vi "Test_PromoteElementAtTop_NoChange.vi"(8 "error in (no error)":errorcluster, 11 "TestCase in":refnum<class "TestArrayExtensions.lvclass">) -> (0 "error out":errorcluster, 3 "TestCase out":refnum<class "TestArrayExtensions.lvclass">)   [LabVIEW 2015, in "TestArrayExtensions.lvclass"]
uses:
  TestArrayExtensions.lvclass
  Promote Element (I32).vi
  <vilib>/addons/_JKI Toolkits/VI Tester/TestCase.llb/TestCase.lvclass
  ArrayExtensions.lvlib
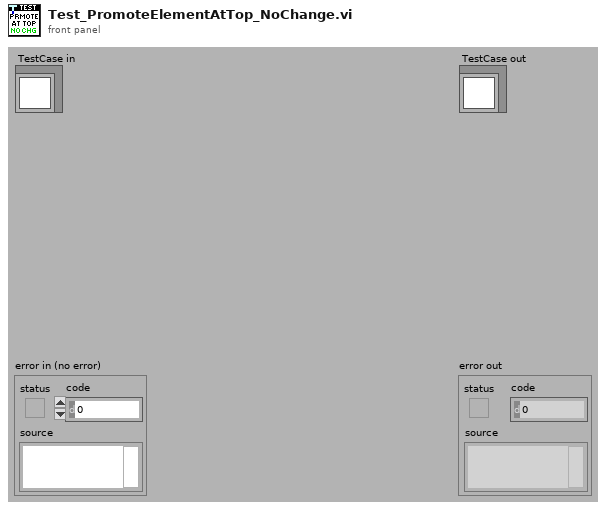
[diagram p1: front panel]
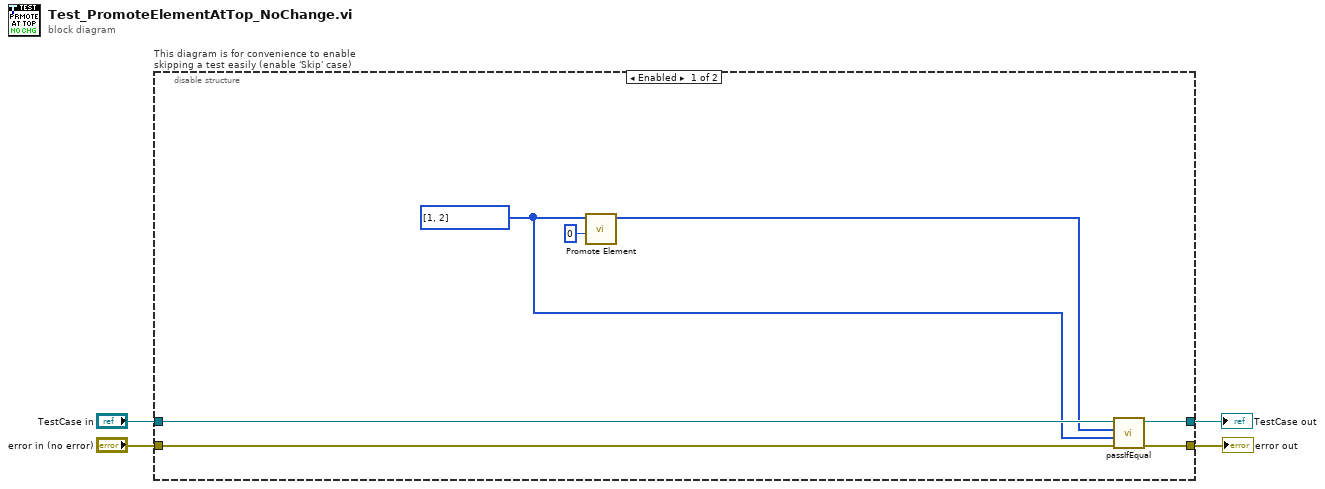
[diagram p0: block diagram]
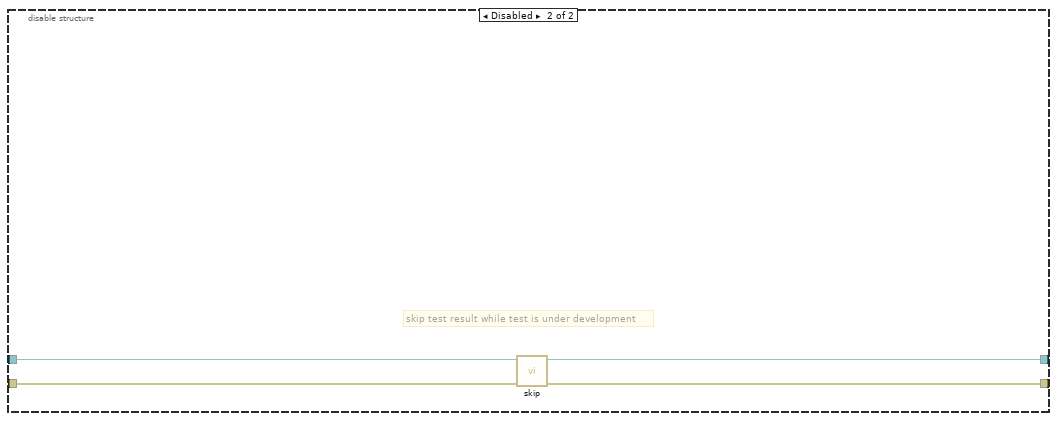
[diagram p2: hidden frame]
diagram:
  n1 = disable-structure "This diagram is for convenience to enable skipping a test easily (enable 'Skip' case)" shown="Enabled" {
    disable-tunnel: "TestCase in" -> [w11 w15]
    disable-tunnel: [w10 w13] -> w1
    disable-tunnel: [w9 w14] -> w3
    disable-tunnel: "error in (no error)" -> [w8 w12]
    frame Enabled {
      w5 = i32[] [1, 2]
      n2 = call-poly "Promote Element.vi"("Index to Promote"=0, "Array In"=w5) -> ("Array Out"=w6:i32[])  [unwired: 9 in]
      n3 = call-dynamic "passIfEqual.vi"("error in (no error)"=w8, "y"=w5, "x"=w6, "TestCase in"=w11) -> ("error out"=w9:errorcluster, "TestCase out"=w10:refnum<class "TestArrayExtensions.lvclass">)  [unwired: 6 in]
    }
    frame Disabled {
      # "skip test result while test is under development"
      n4 = call <vilib>:"skip.vi"("error in (no error)"=w12, "TestCase in"=w15) -> ("error out"=w14:errorcluster, "TestCase out"=w13:refnum<class "TestArrayExtensions.lvclass">)  [unwired: 8 in]
    }
  }
  "error out" <- w3
  "TestCase out" <- w1
